vi "RSZVL_MeasurePulsedPower.vi"(0 "VISA resource name":refnum<visa-resource-name>="SpecAn_1", 1 "Center Freq.":dbl=1000000000.0 caption="Center Freq. (Hz)", 2 "Sweep Time":dbl=50.0 caption="Sweep Time (mS)", 3 "Ref. Level":dbl caption="Ref. Level (dBm)", 4 "Measurement Type":enum16{"RMS Power", "Peak Power"}(ring)=enum."Peak Power", 5 "error in (no error)":errorcluster {"code" format="%.0x"}, 6 "Trigger Offset":dbl=-10.0 caption="Trigger Offset (mS)", 7 "Left Limit":dbl=5.0 caption="Left Limit  (mS)", 8 "Trigger Level":dbl=-20.0 caption="Trigger Level (dBm)", 9 "Right Limit":dbl=6.0 caption="Right Limit  (mS)", 10 "Route Names":string[](array[string]), 12 "Calibration Enabled":bool) -> (14 "Peak Power Calibrated":dbl=-9.89595207905 caption="Measured Power Calibrated", 16 "Peak Power Raw":dbl=-9.89595207905 caption="Measured Power Raw", 19 "error out":errorcluster {"code" format="%.0x"})   [LabVIEW 2015]
doc: "This Vi is used for Measuring RF Power that is pulsed, using R&S ZVL Spectrum Analyzer.\nUsing this technique Power Over-shoot can be measured or avoided to measure true power of pulse.\n\n1- Spec. An is placed in Zero Span mode and the center freq is at the frequency of the RF signal\n2- Set Sweep Time, Ref. Level and Trigger settings to get at least one pulse\n3- Adjust left & Right Limit lines anywher on the pulse, Left Limit at 0 will be at the start of the pulse\n4- Power between the Left & Right limit Lines is measured"
panel:
  # "Measure Pulse Power"
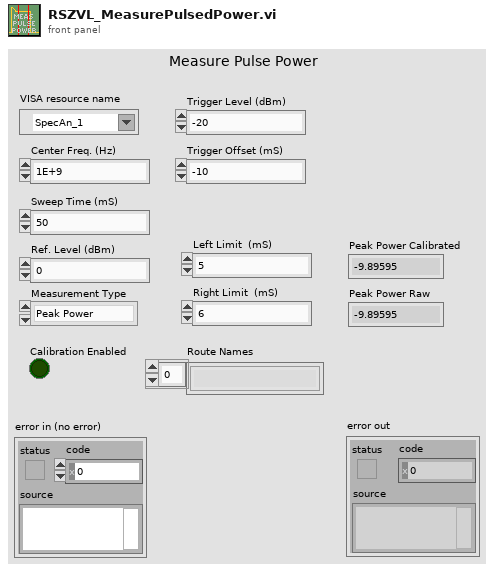
[diagram p1: front panel]
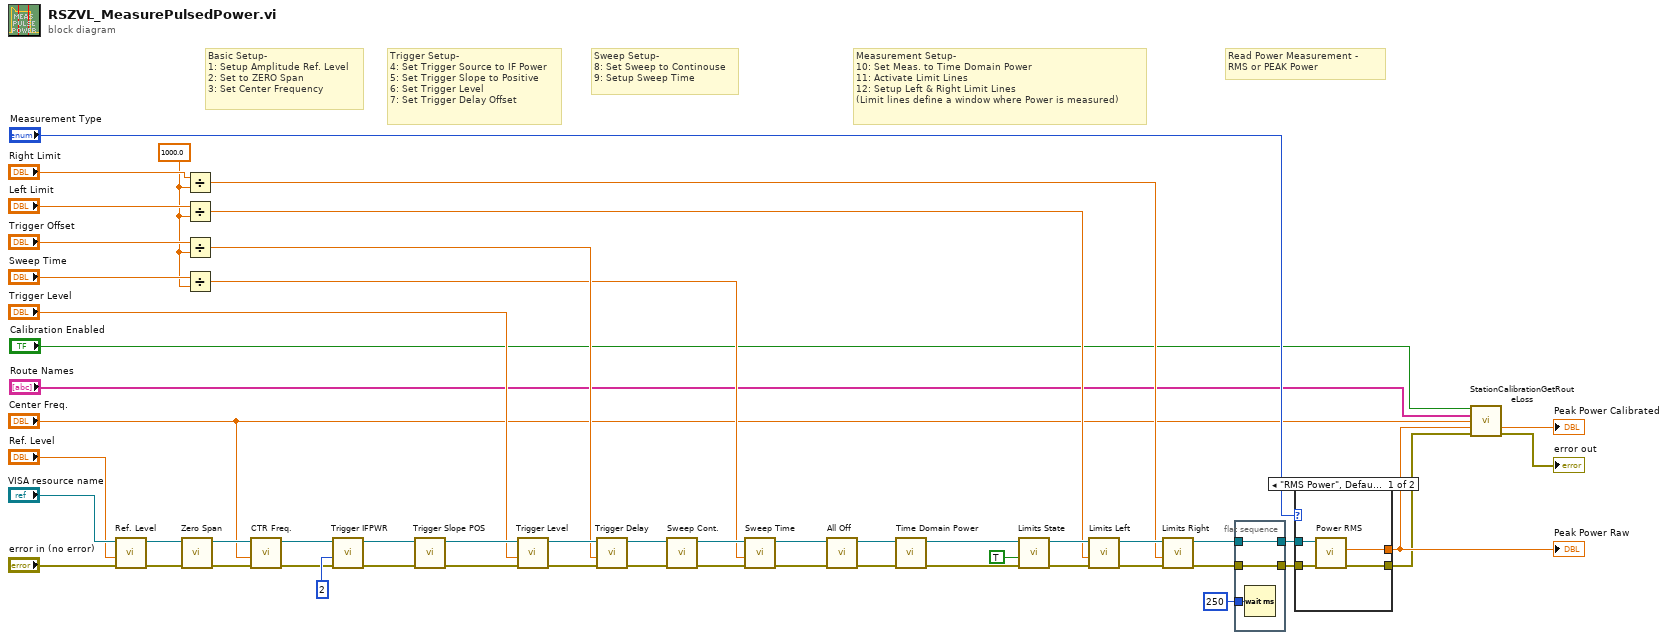
[diagram p0: block diagram]
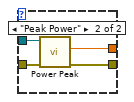
[diagram p2: hidden frame]
diagram:
  w19 = 1000.0 ("y")
  # "Read Power Measurement -\nRMS or PEAK Power"
  # "Measurement Setup-\n10: Set Meas. to Time Domain Power\n11: Activate Limit Lines\n12: Setup Left & Right Limit Lines\n(Limit lines define a window where Power is measured)"
  # "Sweep Setup-\n8: Set Sweep to Continouse\n9: Setup Sweep Time"
  # "Trigger Setup-\n4: Set Trigger Source to IF Power\n5: Set Trigger Slope to Positive\n6: Set Trigger Level\n7: Set Trigger Delay Offset"
  # "Basic Setup-\n1: Setup Amplitude Ref. Level\n2: Set to ZERO Span\n3: Set Center Frequency"
  n1 = call "Ref. Level"("error in (no error)"="error in (no error)", "Input Double"="Ref. Level", "instrument handle"="VISA resource name") -> ("error out"=w33:errorcluster, "instrument handle out"=w32:refnum<visa-resource-name>)  [unwired: 7 in]
  n2 = call "Zero Span"("error in (no error)"=w33, "instrument handle"=w32) -> ("error out"=w53:errorcluster, "instrument handle out"=w54:refnum<visa-resource-name>)  [unwired: 8 in]
  n3 = Divide(x="Right Limit", y=w19) -> (x/y=w20:dbl)
  n4 = Divide(x="Left Limit", y=w19) -> (x/y=w21:dbl)
  n5 = Divide(x="Trigger Offset", y=w19) -> (x/y=w38:dbl)
  n6 = Divide(x="Sweep Time", y=w19) -> (x/y=w37:dbl)
  n7 = call "CTR Freq."("error in (no error)"=w53, "Input Double"="Center Freq.", "instrument handle"=w54) -> ("error out"=w43:errorcluster, "instrument handle out"=w44:refnum<visa-resource-name>)  [unwired: 7 in]
  n8 = call "Trigger IFPWR"("error in (no error)"=w43, "Input I32"=2, "instrument handle"=w44) -> ("error out"=w46:errorcluster, "instrument handle out"=w47:refnum<visa-resource-name>)  [unwired: 7 in]
  n9 = call "Trigger Slope POS"("error in (no error)"=w46, "instrument handle"=w47) -> ("error out"=w41:errorcluster, "instrument handle out"=w42:refnum<visa-resource-name>)  [unwired: 8 in]
  n10 = call "Trigger Level"("error in (no error)"=w41, "Input Double"="Trigger Level", "instrument handle"=w42) -> ("error out"=w49:errorcluster, "instrument handle out"=w50:refnum<visa-resource-name>)  [unwired: 7 in]
  n11 = call "Trigger Delay"("error in (no error)"=w49, "Input Double"=w38, "instrument handle"=w50) -> ("error out"=w39:errorcluster, "instrument handle out"=w40:refnum<visa-resource-name>)  [unwired: 7 in]
  n12 = call "Sweep Cont."("error in (no error)"=w39, "instrument handle"=w40) -> ("error out"=w51:errorcluster, "instrument handle out"=w52:refnum<visa-resource-name>)  [unwired: 8 in]
  n13 = call "Sweep Time"("error in (no error)"=w51, "Input Double"=w37, "instrument handle"=w52) -> ("error out"=w15:errorcluster, "instrument handle out"=w16:refnum<visa-resource-name>)  [unwired: 7 in]
  n14 = call "All Off"("error in (no error)"=w15, "instrument handle"=w16) -> ("error out"=w13:errorcluster, "instrument handle out"=w14:refnum<visa-resource-name>)  [unwired: 8 in]
  n15 = call "Time Domain Power"("error in (no error)"=w13, "instrument handle"=w14) -> ("error out"=w28:errorcluster, "instrument handle out"=w27:refnum<visa-resource-name>)  [unwired: 8 in]
  n16 = call "Limits State"("error in (no error)"=w28, "Input Boolean"=TRUE, "instrument handle"=w27) -> ("error out"=w25:errorcluster, "instrument handle out"=w26:refnum<visa-resource-name>)  [unwired: 7 in]
  n17 = call "Limits Left"("error in (no error)"=w25, "Input Double"=w21, "instrument handle"=w26) -> ("error out"=w24:errorcluster, "instrument handle out"=w23:refnum<visa-resource-name>)  [unwired: 7 in]
  n18 = call "Limits Right"("error in (no error)"=w24, "Input Double"=w20, "instrument handle"=w23) -> ("error out"=w10:errorcluster, "instrument handle out"=w12:refnum<visa-resource-name>)  [unwired: 7 in]
  n19 = flat-sequence {
    tunnel: w12 -> [w57]
    tunnel: [w57] -> w11
    tunnel: w10 -> [w56]
    tunnel: [w56] -> w9
    tunnel: u32 250 ("Input I32") -> [w55]
    frame #0 {
      n20 = Wait (ms)(milliseconds to wait=w55) -> ()  [unwired: 1 out]
    }
  }
  n21 = case shown="\"RMS Power\", Default" "Measurement Type" {
    tunnel: w9 -> [w61 w64]
    tunnel: w11 -> [w60 w65]
    tunnel: [w59 w62] -> w3
    tunnel: [w58 w63] -> w4
    frame "RMS Power", Default {
      n22 = call "Power RMS"("error in (no error)"=w61, "instrument handle"=w60) -> ("error out"=w59:errorcluster, "Output Double"=w58:dbl)  [unwired: 7 in, 1 out]
    }
    frame "Peak Power" {
      n23 = call "Power Peak"("error in (no error)"=w64, "instrument handle"=w65) -> ("error out"=w62:errorcluster, "Output Double"=w63:dbl)  [unwired: 7 in, 1 out]
    }
  }
  "Peak Power Raw" <- w4
  n24 = call "StationCalibrationGetRouteLoss.vi"("Calibration Enabled"="Calibration Enabled", "Route Names"="Route Names", "Frequency"="Center Freq.", "Power Level"=w4, "error in (no error)"=w3) -> ("Adjusted Power Level"=→"Peak Power Calibrated":dbl, "error out"=→"error out":errorcluster)  [unwired: 7 in, 2 out]
